vi "Dispense FN - OFF - State Status (SubVI).vi"(1 "Measured Mass (g)":dbl, 2 "State Change Pulse":bool, 3 "Level Slope?":bool, 5 "Static Setpoint (g)":dbl, 7 "Elapsed Time (s)":dbl, 9 "Max Drain Complete?":bool) -> (14 "ON Signal":bool, 19 "Complete":bool)   [LabVIEW 2009]
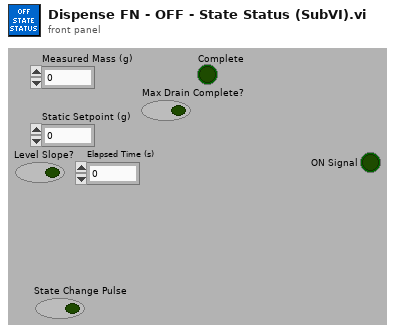
[diagram p1: front panel]
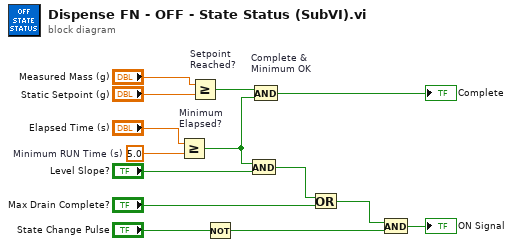
[diagram p0: block diagram]
diagram:
  w11 = 5.0  # Minimum RUN Time (s)
  n1 = Greater Or Equal? "Minimum\nElapsed?"(x="Elapsed Time (s)", y=w11) -> (x >= y?=w7:bool)
  n2 = Greater Or Equal? "Setpoint\nReached?"(x="Measured Mass (g)", y="Static Setpoint (g)") -> (x >= y?=w12:bool)
  n3 = Not(x="State Change Pulse") -> (.not. x?=w9:bool)
  n4 = And(x=w7, y="Level Slope?") -> (x .and. y?=w2:bool)
  n5 = And "Complete &\nMinimum OK"(x=w12, y=w7) -> (x .and. y?=→"Complete":bool)
  n6 = Or(x=w2, y="Max Drain Complete?") -> (x .or. y?=w1:bool)
  n7 = And(x=w1, y=w9) -> (x .and. y?=→"ON Signal":bool)
